vi "controlLinealSimple.vi"() -> ()   [LabVIEW 2021]
panel:
  out "Control":T1(graph)
  out "X2":dynamicdata(graph)
  out "SeñalU":cluster{"X":dbl[], "Y":dbl[]}[](graph)
  out "Error":cluster{"X":dbl[], "Y":dbl[]}[](graph)
  out "X1":dynamicdata(graph)
  in  "stop":bool
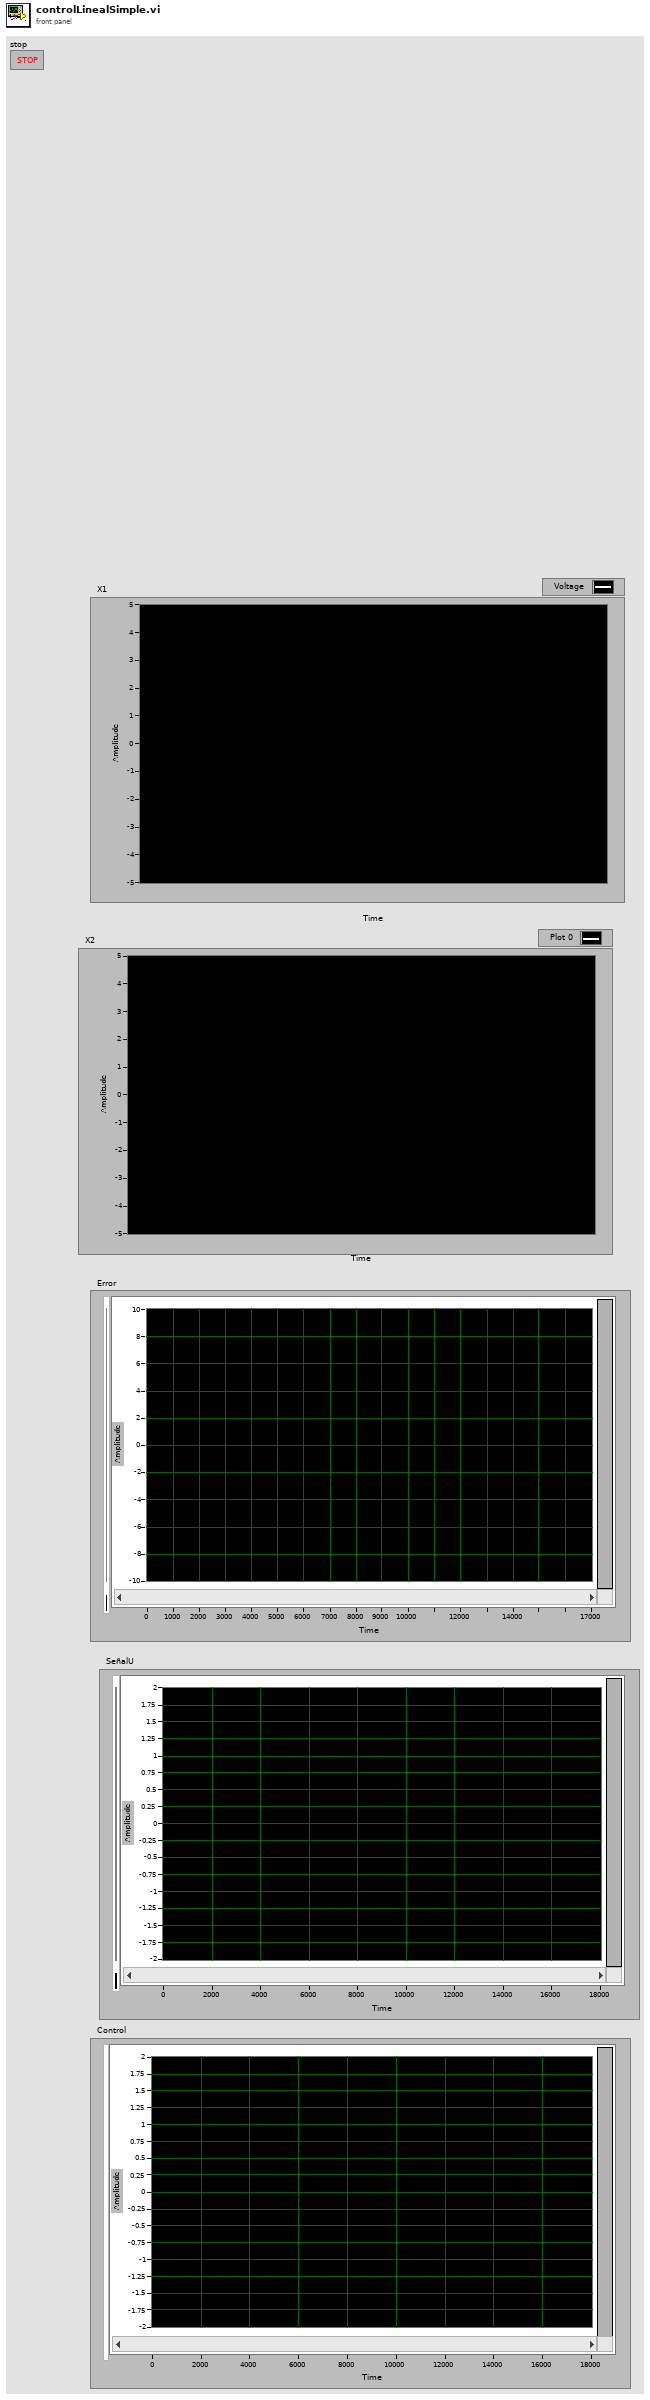
[diagram p1: front panel]
types:
  T1 = cluster{"XY Graph":cluster{"X":dbl[], "Y":dbl[]}[], "XY Graph":cluster{"X":dbl[], "Y":dbl[]}[]}
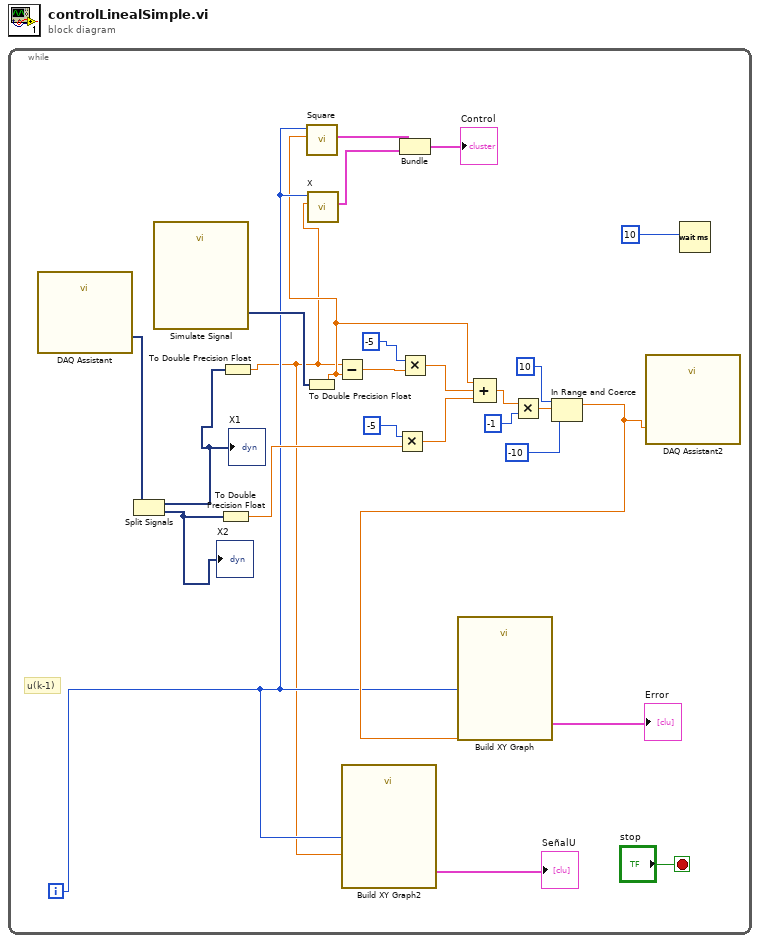
[diagram p0: block diagram]
diagram:
  n1 = while {
    i -> [w3]
    stop <- "stop" stop-if-true
    # "u(k-1)"
    n2 = call "DAQ Assistant"() -> ("data"=w22:dynamicdata)  [unwired: 17 in, 2 out]
    n3 = Split Signals(w22) -> (w20:dynamicdata, w21:dynamicdata)  [unwired: 2 in]
    "X1" <- w20
    "X2" <- w21
    n4 = call "Simulate Signal"() -> ("Square"=w4:dynamicdata)  [unwired: 14 in, 1 out]
    n5 = To Double Precision Float(number=w21) -> (double precision float=w14:dbl)
    n6 = To Double Precision Float(number=w20) -> (double precision float=w1:dbl)
    n7 = To Double Precision Float(number=w4) -> (double precision float=w2:dbl)
    n8 = call "Square"("Y Input"=w2, "X Input"=w3) -> ("XY Graph"=w5:cluster{"X":dbl[], "Y":dbl[]}[])  [unwired: 8 in, 1 out]
    n9 = call "X"("Y Input"=w1, "X Input"=w3) -> ("XY Graph"=w6:cluster{"X":dbl[], "Y":dbl[]}[])  [unwired: 8 in, 1 out]
    n10 = Subtract(x=w1, y=w2) -> (x-y=w15:dbl)
    n11 = call "Build XY Graph2"("Y Input"=w1, "X Input"=w3) -> ("XY Graph"=→"SeñalU":cluster{"X":dbl[], "Y":dbl[]}[])  [unwired: 8 in, 1 out]
    n12 = Multiply(x=-5, y=w14) -> (x*y=w12:dbl)
    n13 = Bundle("XY Graph"=w5, "XY Graph"=w6) -> (→"Control":T1)  [unwired: 1 in]
    n14 = Multiply(x=-5, y=w15) -> (x*y=w11:dbl)
    n15 = Compound Arithmetic op=ADD(w2, w11, w12) -> (w10:dbl)
    n16 = Multiply(x=w10, y=-1) -> (x*y=w9:dbl)
    n17 = In Range and Coerce(upper limit=10, x=w9, lower limit=-10) -> (coerced(x)=w16:dbl)  [unwired: 1 out]
    n18 = call "Build XY Graph"("Y Input"=w16, "X Input"=w3) -> ("XY Graph"=→"Error":cluster{"X":dbl[], "Y":dbl[]}[])  [unwired: 8 in, 1 out]
    n19 = call "DAQ Assistant2"("data"=w16) -> ()  [unwired: 17 in, 2 out]
    n20 = Wait (ms)(milliseconds to wait=10) -> ()  [unwired: 1 out]
  }
